vi "Problem_2.vi"() -> ()   [LabVIEW 2022 SP3]
uses:
  <vilib>/Utility/file.llb/Read Delimited Spreadsheet (DBL).vi
panel:
  out "Finals Answer w/ pervious values removed":dbl(graph)
  out "array (last n elements first)":dbl[](array[numeric])
  out "Data After Weighted":dbl(graph)
  out "size(s)":i32[](array[numeric])
  out "All Data":dbl[](graph)
  in  "file path (dialog if empty)":path=path "C:/Users/Luisa Guarco/Documents/MATLAB/ME70/Homework #1/SampleTempBoiling.txt"
  in  "stop":bool
  # "Array 2 holds all of the data"
  # "This is what is rotating the data \nin and out"
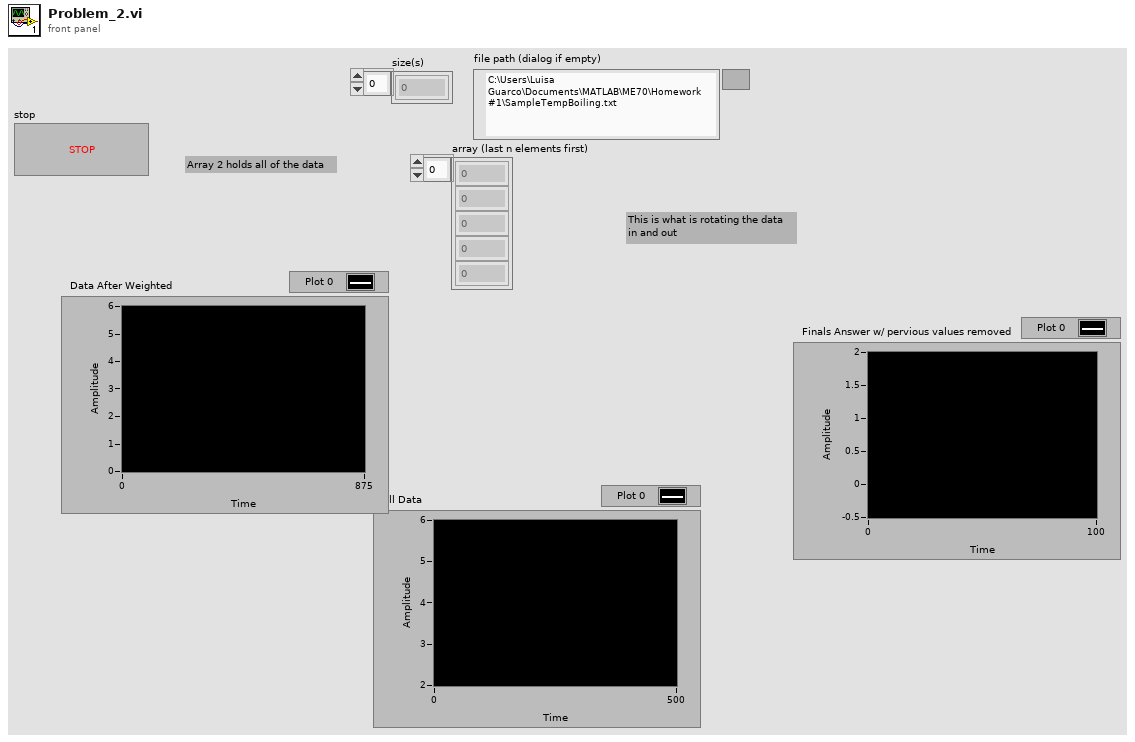
[diagram p1: front panel]
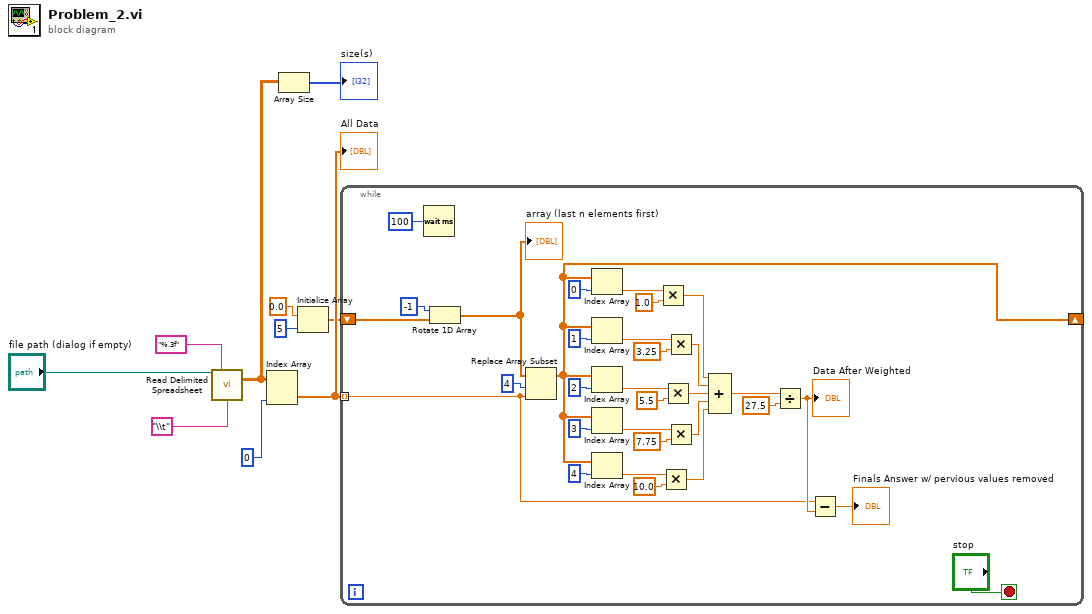
[diagram p0: block diagram]
diagram:
  n1 = call-poly <vilib>:"Read Delimited Spreadsheet.vi"("file path (dialog if empty)"="file path (dialog if empty)", "format (%.3f)"="%.3f", "delimiter (\\t)"="\\t" ("delimiter (\\t)")) -> ("all rows"=w6:dbl[][])  [unwired: 7 in, 5 out]
  n2 = Index Array "Index Array"(array=w6, index (col)=0 ("disabled index (col)")) -> (element=w4:dbl[])  [unwired: 1 in]
  "All Data" <- w4
  n3 = Array Size(array=w6) -> (size(s)=→"size(s)":i32[])
  n4 = Initialize Array(0.0 ("element"), 5 ("dimension size")) -> (w2:dbl[])
  n5 = while {
    tunnel: w4 -> [w12] mode=indexing
    shift-right: [w28] -> _
    shift-left: w2 -> [w29]
    stop <- "stop" stop-if-true
    n6 = Wait (ms)(milliseconds to wait=u32 100 ("millisecond timer value")) -> ()  [unwired: 1 out]
    n7 = Rotate 1D Array(1:w29, 2:-1 ("n")) -> (0:w16:dbl[])
    "array (last n elements first)" <- w16
    n8 = Replace Array Subset(array=w16, new element=w12, index=4) -> (w28:dbl[])
    n9 = Index Array(array=w28, index=0) -> (element=w39:dbl)
    n10 = Index Array(array=w28, index=1) -> (element=w34:dbl)
    n11 = Index Array(array=w28, index=2) -> (element=w33:dbl)
    n12 = Index Array(array=w28, index=3) -> (element=w32:dbl)
    n13 = Index Array(array=w28, index=4) -> (element=w31:dbl)
    n14 = Multiply(x=w39, y=1.0) -> (x*y=w27:dbl)
    n15 = Multiply(x=w31, y=10.0) -> (x*y=w23:dbl)
    n16 = Multiply(x=w33, y=5.5) -> (x*y=w25:dbl)
    n17 = Multiply(x=w34, y=3.25) -> (x*y=w26:dbl)
    n18 = Multiply(x=w32, y=7.75) -> (x*y=w24:dbl)
    n19 = Compound Arithmetic op=ADD(w27, w26, w25, w24, w23) -> (w22:dbl)
    n20 = Divide(x=w22, y=27.5) -> (x/y=w13:dbl)
    "Data After Weighted" <- w13
    n21 = Subtract(x=w12, y=w13) -> (x-y=→"Finals Answer w/ pervious values removed":dbl)
  }
